vi "AutoOneBallCollector.vi"(8 "error in (no error)":errorcluster) -> (0 "error out":errorcluster)   [LabVIEW 2013]
uses:
  AutoStates.ctl
  AutoMode.ctl
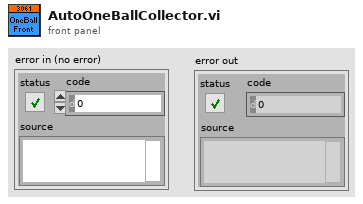
[diagram p1: front panel]
types:
  T1 = typedef "AutoStates.ctl" = enum16{"Init", "LowerArm", "CheckGoal", "Collect", "StopCollect", "RaiseServo", "Drive", "Wait", "ShootCollectorUp", "RaiseArm", "ShootCollectorDown", "Rotate1", "Rotate2", "Stop"}
  T2 = typedef "AutoMode.ctl" = enum16{"OneBallFront", "OneBallCollector", "TwoBallNormal", "TwoBallHot"}
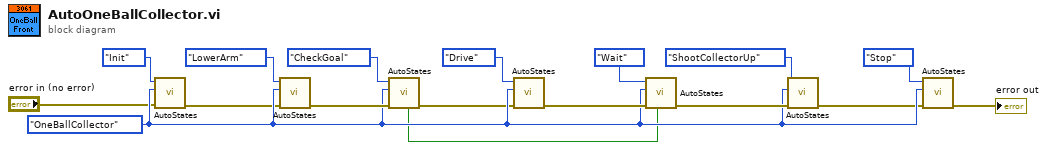
[diagram p0: block diagram]
diagram:
  w8 = AutoMode."OneBallCollector" ("AutoMode")
  n1 = call "AutoStates.vi"("error in (no error)"="error in (no error)", "AutoMode"=w8, "AutoState"=AutoStates."Init") -> ("error out"=w3:errorcluster)  [unwired: 7 in, 1 out]
  n2 = call "AutoStates.vi"("error in (no error)"=w3, "AutoMode"=w8, "AutoState"=AutoStates."LowerArm") -> ("error out"=w14:errorcluster)  [unwired: 7 in, 1 out]
  n3 = call "AutoStates.vi"("error in (no error)"=w14, "AutoMode"=w8, "AutoState"=AutoStates."CheckGoal") -> ("error out"=w2:errorcluster, "Hot?"=w6:bool)  [unwired: 7 in]
  n4 = call "AutoStates.vi"("error in (no error)"=w2, "AutoMode"=w8, "AutoState"=AutoStates."Drive") -> ("error out"=w9:errorcluster)  [unwired: 7 in, 1 out]
  n5 = call "AutoStates.vi"("WasHot?"=w6, "error in (no error)"=w9, "AutoMode"=w8, "AutoState"=AutoStates."Wait") -> ("error out"=w10:errorcluster)  [unwired: 6 in, 1 out]
  n6 = call "AutoStates.vi"("error in (no error)"=w10, "AutoMode"=w8, "AutoState"=AutoStates."ShootCollectorUp") -> ("error out"=w1:errorcluster)  [unwired: 7 in, 1 out]
  n7 = call "AutoStates.vi"("error in (no error)"=w1, "AutoMode"=w8, "AutoState"=AutoStates."Stop") -> ("error out"=→"error out":errorcluster)  [unwired: 7 in, 1 out]
